vi "config-ICC.vi"() -> ()   [LabVIEW 2024]
uses:
  controls/controller.ctl
  controls/sched-cluster.ctl
  controls/UiScheduleTimestamp.ctl
  controls/UiDeviceSensorParams.ctl
  controls/UiDeviceSensorEquality.ctl
  controls/device-mode.ctl
  controls/UiStepBuilder.ctl
  controls/type.step-builder.ctl
  <vilib>/Utility/miscctls.llb/LVPointTypeDef.ctl
  controls/enumVarCtrlIO.ctl
  controls/enum.io.type.ctl
  controls/enum.io.mode.ctl
  <vilib>/Utility/error.llb/DialogType.ctl
  controls/state-engine.ctl
  <vilib>/Utility/libraryn.llb/Create Directory Recursive.vi
  globals/globals-engine.vi
panel:
  out "procNameID":string
  in  "Ctrl Reload":bool
  in  "Help Page":bool
  in  "Tab Control":enum32{"Main", "Manual Activation", "Help"}(tab)
  in  "Ctrl Save":bool
  in  "Controller":T1={"Schedular"={"sched-mode"=enum."Hourly", "sched-pairs"=[]}, "Sensor"={"Input"="INPUT:", "Comparison"=">=", "Setpoint"=0.0}, "Outputs"=[], "Interval"=0, "Timeout"=1, "Mode"=enum."On"} caption="Device Setup" {"Schedular"."sched-pairs"."start" format="%<%H:%M %d/%m>T"; "Schedular"."sched-pairs"."stop" format="%<%H:%M %d/%m>T"; "Timeout" min=1}
  in  "SEC":u16(ring)=1 caption="Section" items=["H1"]
  in  "Manual.Activation":bool
  in  "DEV":u16(ring)=1 caption="Device" items=["CNETFOG", "CO2", "COOLFAN", "FAC_VENT", "Fan1", "Fan2", "Fan3", "PBRDIGEST", "SCREEN", "WETWALL"]
  in  "Cluster":T7={"Send"=FALSE, "Timeout"=10, "State"=FALSE} {"Timeout" min=1 step=1}
  in  "Manual.Return":bool
  in  "Manual.Return 2":bool
  out "NewDevice":string
  in  "Data Changed?":bool=TRUE
  in  "DEV Reload":bool
  in  "SEC Reload":bool
  out "dir name":string="ICC"
  out "Flow Steps":T8[](array[typedef])
  out "event counter":i32
  in  "DEV Set Strings":bool
  in  "SEC Set Strings":bool
  # "Pulse [sec]"
  # "Period [sec]"
  # "Sensor"
  # "Scheduler"
  # "Note: Timeout value must be above zero."
  # "Indoor Climate Control Configurator\n\nFor devices required pulse activation set \nPulse Width parameter greater then zero (and less then Period).\n\nFor devices required constant ON signal set \nPulse Width parameter greater then Period value."
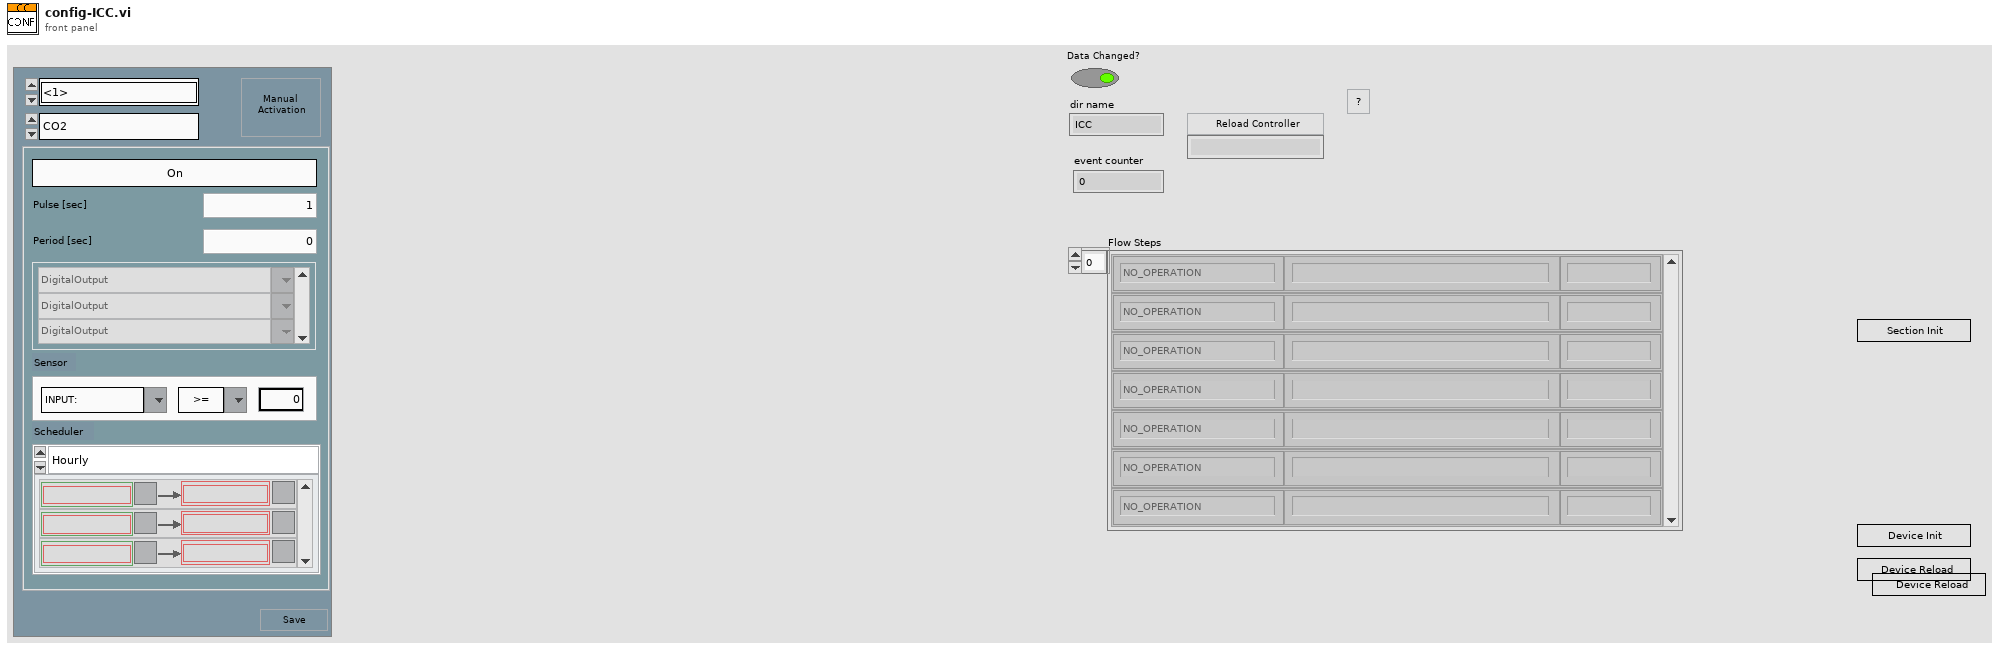
[diagram p1: front panel]
types:
  T1 = typedef "controller.ctl" = cluster{"Schedular":T2, "Sensor":T4, "Outputs":string[], "Interval":u32, "Timeout":u16, "Mode":T6}
  T2 = typedef "sched-cluster.ctl" = cluster{"sched-mode":enum16{"Hourly", "Daily", "Weekly", "Date"}, "sched-pairs":cluster{"start":T3, "stop":T3}[]}
  T3 = typedef "UiScheduleTimestamp.ctl" = timestamp
  T4 = typedef "UiDeviceSensorParams.ctl" = cluster{"Input":string, "Comparison":T5, "Setpoint":dbl}
  T5 = typedef "UiDeviceSensorEquality.ctl" = string
  T6 = typedef "device-mode.ctl" = enum16{"On", "Off", "Sense", "Sched", "Sched AND Sense", "Sched OR Sense"}
  T7 = cluster{"Send":bool, "Timeout":u16, "State":bool}
  T8 = typedef "UiStepBuilder.ctl" = cluster{"Step Function":T9, "ParamString":string, "Step Label":string}
  T9 = typedef "type.step-builder.ctl" = enum16{"NO_OPERATION", "DELAY-JUMP", "DELAY", "JUMP", "COMPLETE", "SCHEDULER", "IRR-CHECK", "UNIT-CHECK", "UNIT-SAMPLE", "UNIT-DOSE", "LOG-REPORT", "LOG-MESSAGE", "IO-READ", "IO-READ-MANY", "IO-WRITE", "IO-COMPARE-OUT", "IO-COMPARE-IN", "PROC-START", "PROC-STOP", "PROC-LOAD", "PROC-IS-COMPLETED", "RECORD-MOVE", "GET-RH", "GET-UV", "GET-WD", "GET-WS", "OCS-CHECK", "OCS-RECORD"}
  T10 = typedef "LVPointTypeDef.ctl" = cluster{"Horizontal":i16, "Vertical":i16}
  T11 = typedef "enum.io.type.ctl" = enum16{"Type", "DI", "DO", "AI", "AO", "VL", "BUF"}
  T12 = typedef "enumVarCtrlIO.ctl" = enum16{"IO Get By Key", "IO List Configs", "IO Add By Key", "IO Modify Value By Key", "IO Modify Calib By Key", "IO Modify ADDR By Key", "IO Modify Mode By Key", "IO Modify Type By Key", "IO Modify Name By Key", "IO Remove By Key", "IO Remove All"}
  T13 = cluster{"state":bool, "timeout":u16, "Name":string}
  T14 = typedef "state-engine.ctl" = enum16{"ENG.NO-OP", "ENG.START", "ENG.STOP", "ENG.EXECUTE", "ENG.STATUS", "ENG.EXTERNAL-CALL", "ENG.INIT", "ENG.INIT.VARS", "ENG.INIT.SERIAL", "ENG.LOAD", "ENG.LOAD.SINGLE", "ENG.LOAD.MODULE", "ENG.LOAD.RELOAD", "ENG.LOAD.UNLOAD", "ENG.IO.LOAD", "ENG.IO.SAVE", "ENG.PROC.RELOAD-BY-NAME", "ENG.PROC.START", "ENG.PROC.STOP", "ENG.PROC.INSERT-STEPS", "ENG.PROC.ISRUNNING", "ENG.PROC.PRESET", "ENG.PROC.STATUS", "ENG.PRINT-USER-MSG", "ENG.RIO.SNAPSHOT", "ENG.RIO.AIN-SNAPSHOT-CALIB", "ENG.RIO.DOUT-BY-ADDR", "ENG.RIO.DOUT-BY-NAME", "ENG.RIO.RFS-DELAY-SET-X1", "ENG.RIO.RFS-DELAY-SET-X8", "ENG.RIO.RFS-CYCLES-SET", "ENG.RIO.RFS-CYCLES-GET", "ENG.RIO.RFS-ENABLE", "ENG.EXIT"}
  T15 = enum32{"Invalid", "Standard", "Closed", "Hidden", "Minimized", "Maximized"}
  T16 = typedef "enum.io.mode.ctl" = enum16{"Mode", "RIO", "SIM"}
  T17 = typedef "IONode.ctl" = cluster{"ADDR":T18, "Label":string, "Type":T11, "Mode":T16, "Value":string, "Tags":string, "calibration":T19[]}
  T18 = typedef "type.address.ctl" = u16
  T19 = typedef "typeXyPoint.ctl" = cluster{"X":dbl, "Y":dbl}
  T20 = typedef "DialogType.ctl" = u16
  T21 = cluster{"Boolean State":bool, "Ch":u8, "Address":u8, "Timeout":u8}
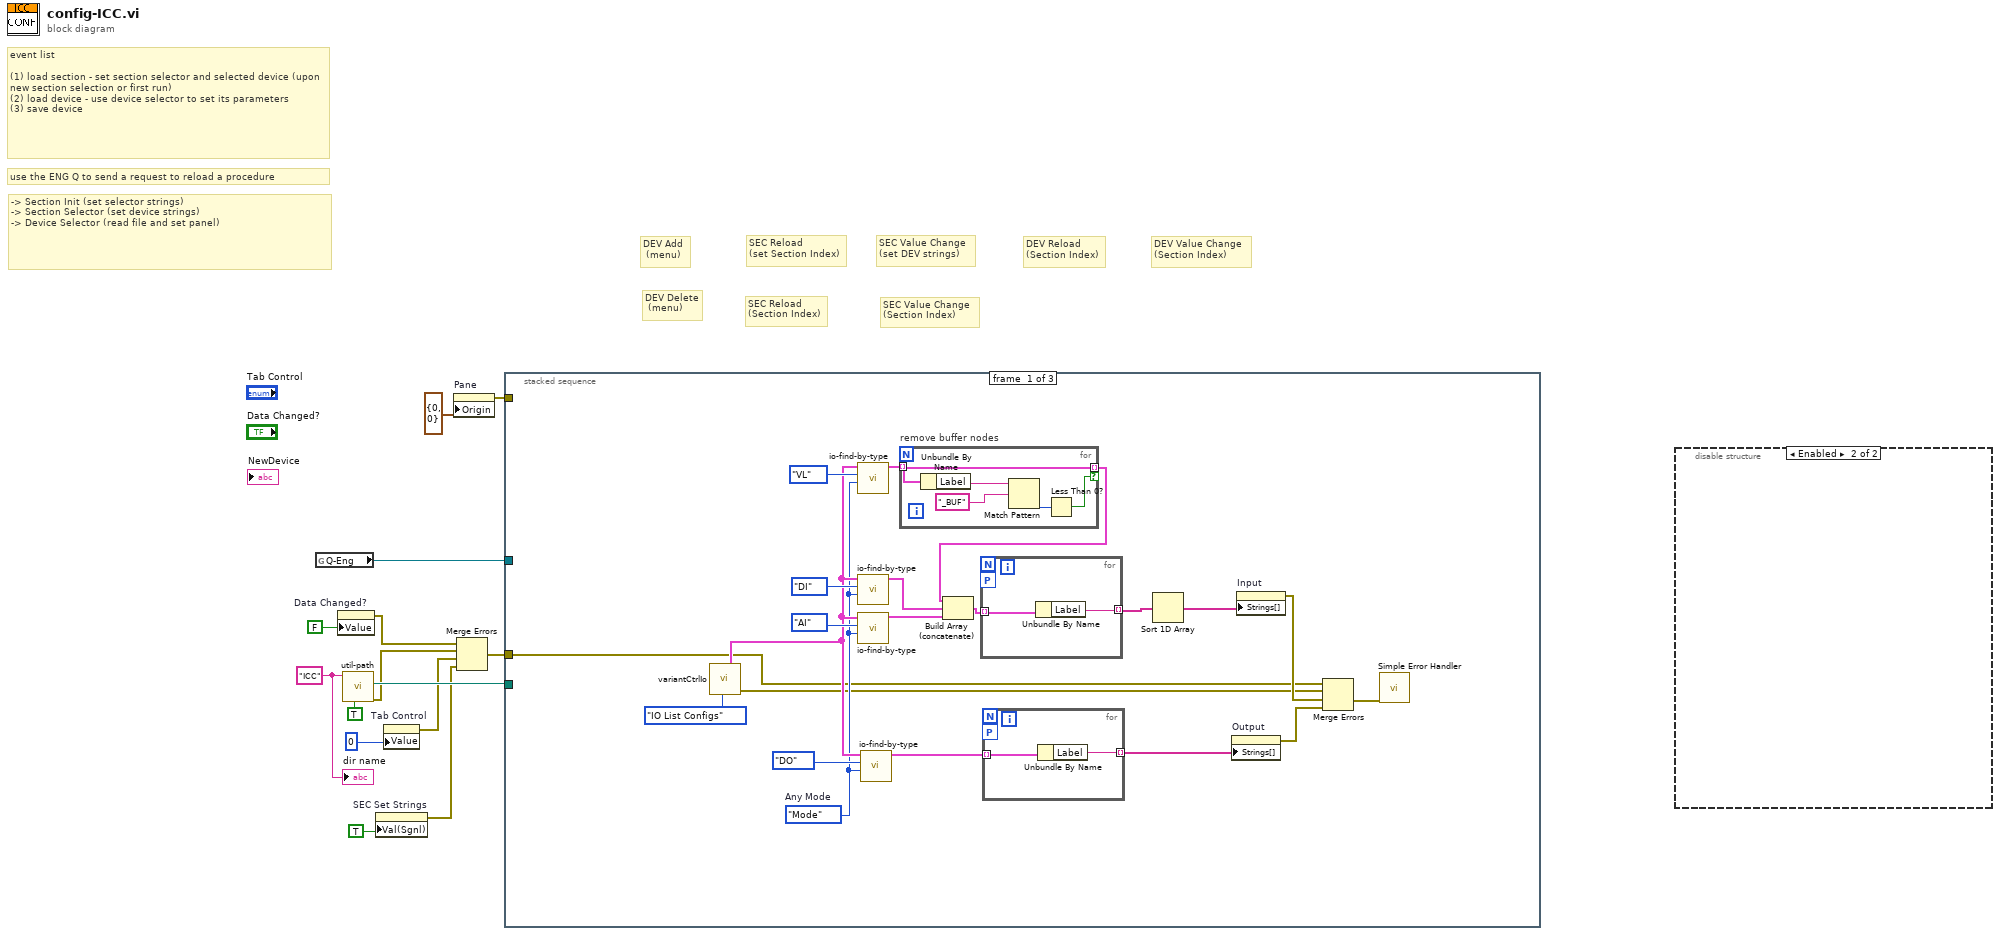
[diagram p0: block diagram]
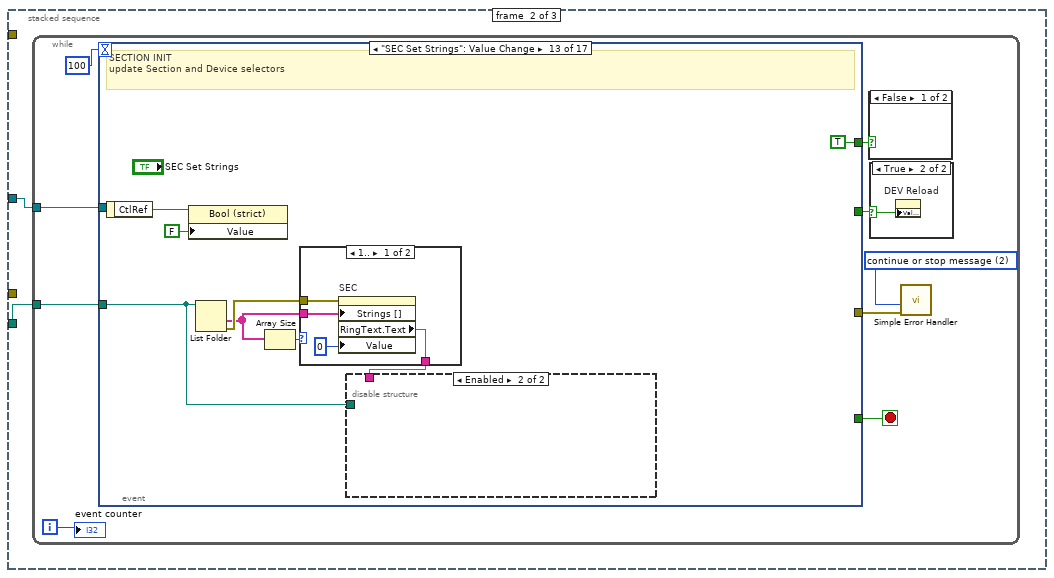
[diagram p3: hidden frame]
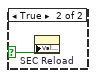
[diagram p5: hidden frame]
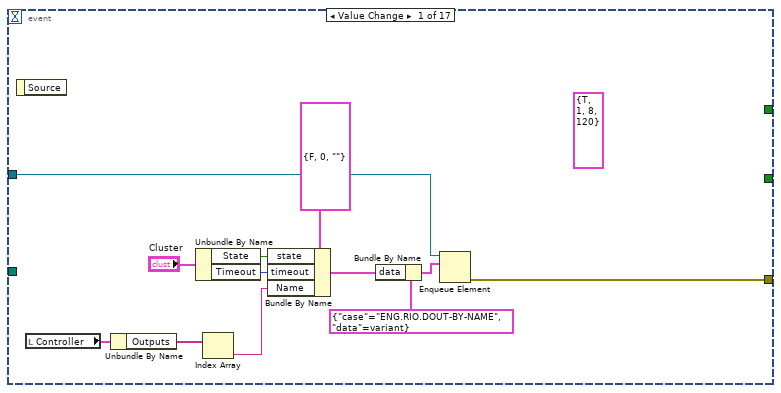
[diagram p6: hidden frame]
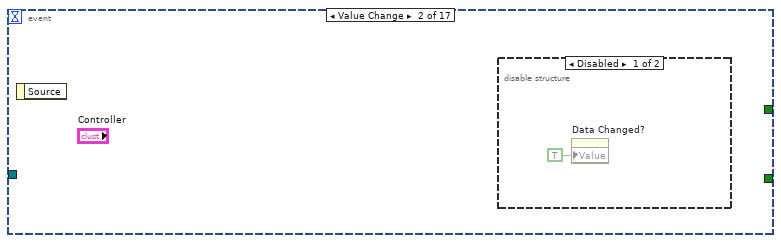
[diagram p7: hidden frame]
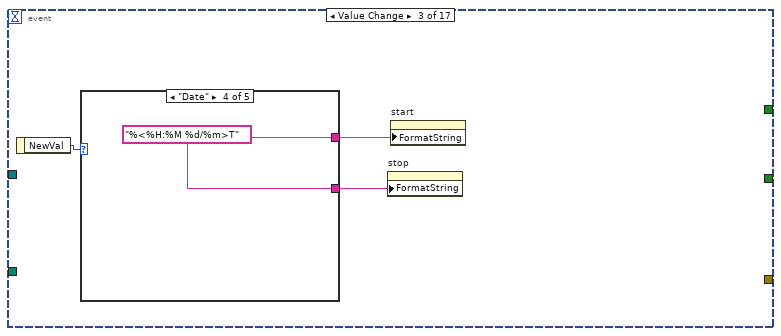
[diagram p9: hidden frame]
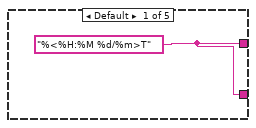
[diagram p10: hidden frame]
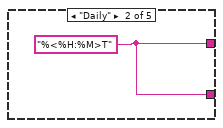
[diagram p11: hidden frame]
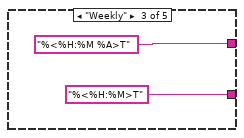
[diagram p12: hidden frame]
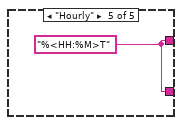
[diagram p13: hidden frame]
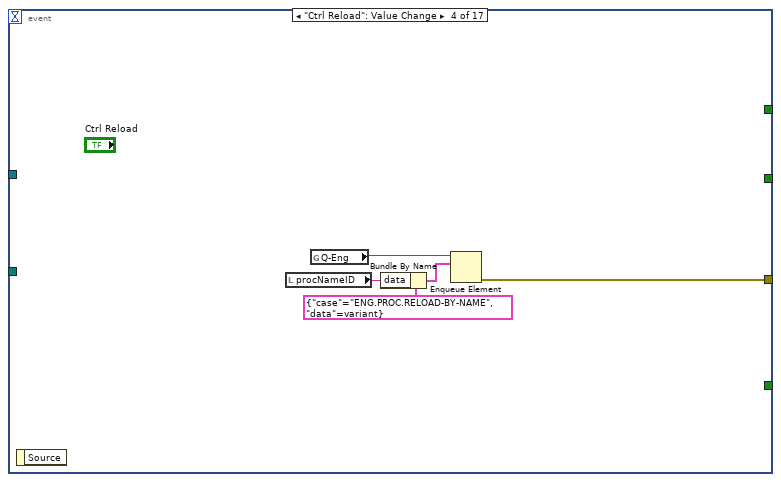
[diagram p14: hidden frame]
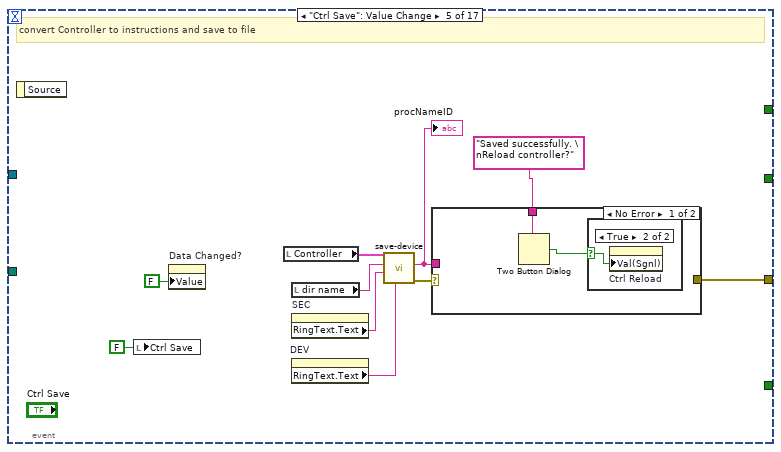
[diagram p15: hidden frame]
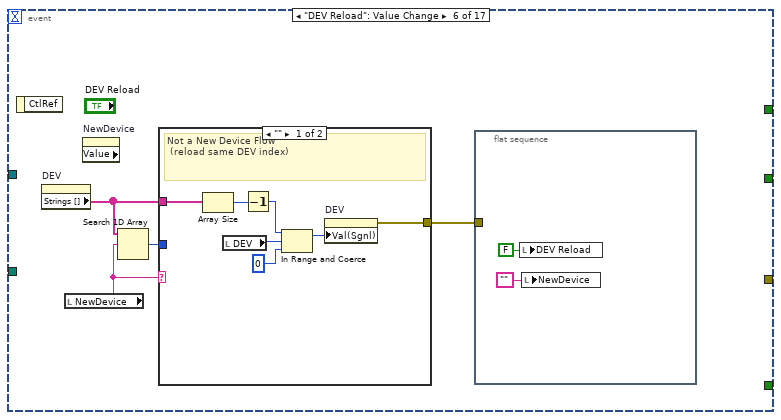
[diagram p18: hidden frame]
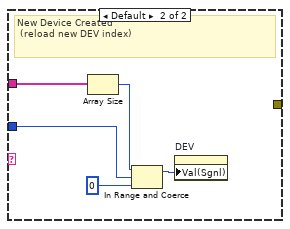
[diagram p19: hidden frame]
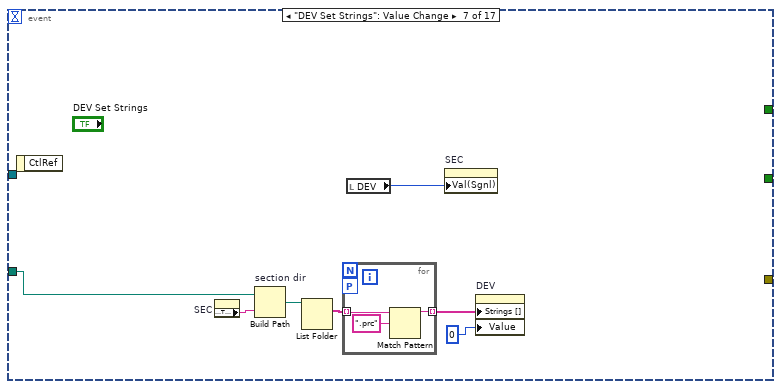
[diagram p20: hidden frame]
diagram:
  w9 = "ICC" ("dir name")
  # "DEV Value Change\n(Section Index)"
  # "SEC Value Change\n(Section Index)"
  # "SEC Reload\n(Section Index)"
  # "DEV Delete\n (menu)"
  # "DEV Reload\n(Section Index)"
  # "DEV Add\n (menu)"
  # "SEC Value Change\n(set DEV strings)"
  # "SEC Reload\n(set Section Index)"
  # "-> Section Init (set selector strings)\n-> Section Selector (set device strings)\n-> Device Selector (read file and set panel)"
  # "use the ENG Q to send a request to reload a procedure"
  # "event list\n\n(1) load section - set section selector and selected device (upon new section selection or first run)\n(2) load device - use device selector to set its parameters \n(3) save device"
  n1 = global read "globals-engine.vi" "Q-Eng"() -> (w7:refnum<queue>)
  n2 = property on="Data Changed?" class="Bool (strict)"("Value"=FALSE ("Data Changed?")) -> (error out=w6:errorcluster)  [unwired: 2 in, 1 out]
  n3 = call "util-path.vi"("Create Folders?(F)"=TRUE, "append path (ie. folder\\filename.*)"=w9) -> ("error out"=w5:errorcluster, "SelectedPath"=w12:path)  [unwired: 5 in, 3 out]
  n4 = property on="SEC Set Strings" class="Bool (strict)"("Val(Sgnl)"=TRUE ("Section Load")) -> (error out=w3:errorcluster)  [unwired: 2 in, 1 out]
  n5 = property on="Tab Control" class="TabCtl (strict)"("Value"=0) -> (error out=w4:errorcluster)  [unwired: 2 in, 1 out]
  n6 = property on="Pane" class="Pane"("Origin"=T10 {"Horizontal"=0, "Vertical"=0}) -> (error out=w13:errorcluster)  [unwired: 2 in, 1 out]
  n7 = Merge Errors(w6, w5, w4, w3) -> (w1:errorcluster)
  n8 = stacked-sequence {
    tunnel: w12 -> [_ w46 _]
    tunnel: w13 -> [_ _ _]
    tunnel: w7 -> [_ w45 _]
    tunnel: w1 -> [w15 _ _]
    frame #0 {
      w23 = enum.io.mode."Mode"  # Any Mode
      n9 = call "variantCtrlIo.vi"("menu (Get Param)"=enumVarCtrlIO."IO List Configs" ("menu (get)")) -> ("error out"=w17:errorcluster, "IO Configs List"=w24:T17[])  [unwired: 6 in, 3 out]
      n10 = call "io-find-by-type.vi"("Mode(Any)"=w23, "Type"=enum.io.type."VL" ("type"), "IOConfigs in"=w24) -> ("Search Results"=w22:T17[])  [unwired: 8 in]
      n11 = call "io-find-by-type.vi"("Mode(Any)"=w23, "Type"=enum.io.type."DI" ("type"), "IOConfigs in"=w24) -> ("Search Results"=w32:T17[])  [unwired: 8 in]
      n12 = call "io-find-by-type.vi"("Mode(Any)"=w23, "Type"=enum.io.type."AI" ("type"), "IOConfigs in"=w24) -> ("Search Results"=w31:T17[])  [unwired: 8 in]
      n13 = call "io-find-by-type.vi"("Mode(Any)"=w23, "Type"=enum.io.type."DO" ("type"), "IOConfigs in"=w24) -> ("Search Results"=w27:T17[])  [unwired: 8 in]
      n14 = for "remove buffer nodes" {
        tunnel: w22 -> [w37] mode=indexing
        tunnel: [w37] -> w21 mode=indexing if=w36
        n15 = Unbundle By Name(w37) -> ("Label"=w40:string)
        n16 = Match Pattern(string=w40, regular expression="_BUF") -> (offset past match=w38:i32)  [unwired: 1 in, 3 out]
        n17 = Less Than 0?(x=w38) -> (x < 0?=w36:bool)
      }
      n18 = Build Array (concatenate)(w21, w32, w31) -> (w30:T17[])
      n19 = for {
        tunnel: w30 -> [w44] mode=indexing
        tunnel: [w43] -> w35 mode=indexing
        workers-P: _ -> [_]
        n20 = Unbundle By Name(w44) -> ("Label"=w43:string)
      }
      n21 = for {
        tunnel: w27 -> [w42] mode=indexing
        tunnel: [w41] -> w26 mode=indexing
        workers-P: _ -> [_]
        n22 = Unbundle By Name(w42) -> ("Label"=w41:string)
      }
      n23 = Sort 1D Array(array=w35) -> (sorted array=w20:string[])
      n24 = property on="Output" class="CmbBox"("Strings[]"=w26) -> (error out=w18:errorcluster)  [unwired: 2 in, 1 out]
      n25 = property on="Input" class="CmbBox"("Strings[]"=w20) -> (error out=w19:errorcluster)  [unwired: 2 in, 1 out]
      n26 = Merge Errors(w15, w17, w19, w18) -> (w16:errorcluster)
      n27 = call <vilib>:"Simple Error Handler.vi"("error in (no error)"=w16) -> ()  [unwired: 4 in, 5 out]
    }
    frame #1 {
      n28 = while {
        tunnel: w46 -> [w54]
        tunnel: w45 -> [w47]
        i -> [w53]
        stop <- w55 stop-if-true
        w51 = T20 2 items=["no dialog", "OK message", "continue or stop message", "OK message + warnings", "continue/stop + warnings"] ("type of dialog (OK msg:1)")
        n29 = event shown="[12] \"SEC Set Strings\": Value Change" {
          selector: _ -> [_ _ _ _ _ _ _ _ _ _ _ _ _ _ _ _ _]
          dyn-events: _ -> [_ _ _ _ _ _ _ _ _ _ _ _ _ _ _ _ _]
          timeout: 100 -> [_ _ _ _ _ _ _ _ _ _ _ _ _ _ _ _ _]
          tunnel: [_ _ _ _ _ _ _ _ _ _ _ _ _ _ FALSE w356 w363] -> w55
          tunnel: w54 -> [_ _ _ _ _ _ w117 _ _ _ _ _ w170 w191 w218 _ _]
          tunnel: [w61 _ _ w80 w88 _ _ w128 _ _ _ _ _ _ w216 _ _] -> w52
          tunnel: [_ _ _ _ _ _ _ _ _ _ _ _ TRUE _ w217 _ _] -> w50
          tunnel: [_ _ _ _ _ _ _ _ _ _ _ _ _ w189 _ _ _] -> w49
          tunnel: w47 -> [w58 _ _ _ _ _ _ _ _ _ _ _ _ _ w214 _ _]
          event "Cluster.Send": Value Change {
            (unwired) T21 {"Boolean State"=TRUE, "Ch"=1, "Address"=8, "Timeout"=120} ("digitalPort")
            n30 = event-data() -> ()  [unwired: 1 in, 1 out]
            n31 = local read "Controller"() -> (w62:T1)
            n32 = Unbundle By Name(w62) -> ("Outputs"=w60:string[])
            n33 = Unbundle By Name("Cluster") -> ("State"=w64:bool, "Timeout"=w63:u16)
            n34 = Index Array(array=w60) -> (element=w59:string)  [unwired: 1 in]
            n35 = Bundle By Name(cluster=T13 {"state"=FALSE, "timeout"=0, "Name"=""} ("Cluster"), "state"=w64, "timeout"=w63, "Name"=w59) -> (w66:T13)
            n36 = Bundle By Name(cluster=cluster{"case":T14, "data":variant} {"case"=enum."ENG.RIO.DOUT-BY-NAME", "data"=variant} ("element"), "data"=w66) -> (w68:cluster{"case":T14, "data":variant})
            n37 = Enqueue Element(queue=w58, element=w68) -> (error out=w61:errorcluster)  [unwired: 2 in, 2 out]
          }
          event Value Change {
            n38 = event-data() -> ()  [unwired: 1 in, 1 out]
            n39 = disable-structure shown="Disabled" {
              frame Disabled {
                n40 = property on="Data Changed?" class="Bool (strict)"("Value"=TRUE ("Data Changed?")) -> ()  [unwired: 2 in, 2 out]
              }
              frame Enabled {
              }
            }
          }
          event Value Change {
            n41 = event-data() -> ("NewVal"=w73:enum16{"Hourly", "Daily", "Weekly", "Date"})  [unwired: 1 in]
            n42 = case shown="\"Date\"" w73 {
              tunnel: [w74 w75 "%<%H:%M %A>T" ("Format String") w78 w79] -> w72
              tunnel: [w74 w75 "%<%H:%M>T" ("Format String") w78 w79] -> w71
              frame Default {
                w74 = "%<%H:%M %d/%m>T" ("Format String")
              }
              frame "Daily" {
                w75 = "%<%H:%M>T" ("Format String")
              }
              frame "Weekly" {
              }
              frame "Date" {
                w78 = "%<%H:%M %d/%m>T" ("Format String")
              }
              frame "Hourly" {
                w79 = "%<HH:%M>T" ("Format String")
              }
            }
            n43 = property on="stop" class="AbsTime (strict)"("FormatString"=w71) -> ()  [unwired: 2 in, 2 out]
            n44 = property on="start" class="AbsTime (strict)"("FormatString"=w72) -> ()  [unwired: 2 in, 2 out]
          }
          event "Ctrl Reload": Value Change {
            n45 = event-data() -> ()  [unwired: 1 in, 1 out]
            n46 = local read "procNameID"() -> (w81:string)
            n47 = global read "globals-engine.vi" "Q-Eng"() -> (w84:refnum<queue>)
            n48 = Bundle By Name(cluster=cluster{"case":T14, "data":variant} {"case"=enum."ENG.PROC.RELOAD-BY-NAME", "data"=variant} ("element"), "data"=w81) -> (w83:cluster{"case":T14, "data":variant})
            n49 = Enqueue Element(queue=w84, element=w83) -> (error out=w80:errorcluster)  [unwired: 2 in, 2 out]
          }
          event "Ctrl Save": Value Change {
            # "convert Controller to instructions and save to file"
            n50 = event-data() -> ()  [unwired: 1 in, 1 out]
            n51 = local write "Ctrl Save"(FALSE ("Ctrl Save")) -> ()
            n52 = property on="Data Changed?" class="Bool (strict)"("Value"=FALSE ("Data Changed?")) -> ()  [unwired: 2 in, 2 out]
            n53 = local read "Controller"() -> (w90:T1)
            n54 = local read "dir name"() -> (w91:string)
            n55 = property on="SEC" class="Ring (strict)"() -> ("RingText.Text"=w93:string)  [unwired: 2 in, 2 out]
            n56 = property on="DEV" class="Ring (strict)"() -> ("RingText.Text"=w92:string)  [unwired: 2 in, 2 out]
            n57 = call "save-device.vi"("Proc Name"=w92, "Module Name"=w93, "Base Folder"=w91, "Device"=w90) -> ("error out"=w89:errorcluster, "procNameID"=w85:string)  [unwired: 6 in]
            "procNameID" <- w85
            n58 = case shown="No Error" w89 {
              selector: w89 -> [_ w98]
              tunnel: w85 -> [_ _]
              tunnel: [_ w98] -> w88
              tunnel: "Saved successfully. \nReload controller?" ("message") -> [w96 _]
              frame No Error {
                n59 = Two Button Dialog(message=w96) -> (T button?=w95:bool)  [unwired: 2 in]
                n60 = case shown="True" w95 {
                  selector: w95 -> [_ w97]
                  frame False {
                  }
                  frame True {
                    n61 = property on="Ctrl Reload" class="Bool (strict)"("Val(Sgnl)"=w97) -> ()  [unwired: 2 in, 2 out]
                  }
                }
              }
              frame Error {
              }
            }
          }
          event "DEV Reload": Value Change {
            n62 = event-data() -> ()  [unwired: 1 in, 1 out]
            n63 = property on="DEV" class="Ring (strict)"() -> ("Strings []"=w102:string[])  [unwired: 2 in, 2 out]
            n64 = local read "NewDevice"() -> (w101:string)
            n65 = property on="NewDevice" class="Str" props=["Value"]() -> ()  [unwired: 2 in, 3 out]
            n66 = Search 1D Array(1D array=w102, element=w101) -> (index of element=w100:i32)  [unwired: 1 in]
            n67 = case shown="\"\"" w101 {
              tunnel: w102 -> [w107 w113]
              tunnel: w100 -> [_ w112]
              tunnel: [w106 _] -> w99
              frame "" {
                # "Not a New Device Flow\n (reload same DEV index)"
                n68 = Array Size(array=w107) -> (size(s)=w110:i32)
                n69 = local read "DEV"() -> (w109:u16)
                n70 = Decrement(x=w110) -> (x-1=w105:i32)
                n71 = In Range and Coerce(upper limit=w105, x=w109, lower limit=0) -> (coerced(x)=w108:i32)  [unwired: 1 out]
                n72 = property on="DEV" class="Ring (strict)"("Val(Sgnl)"=w108) -> (error out=w106:errorcluster)  [unwired: 2 in, 1 out]
              }
              frame Default {
                # "New Device Created\n (reload new DEV index)"
                n73 = Array Size(array=w113) -> (size(s)=w115:i32)
                n74 = In Range and Coerce(upper limit=w115, x=w112, lower limit=0) -> (coerced(x)=w114:i32)  [unwired: 1 out]
                n75 = property on="DEV" class="Ring (strict)"("Val(Sgnl)"=w114) -> ()  [unwired: 2 in, 2 out]
              }
            }
            n76 = flat-sequence {
              tunnel: w99 -> [_]
              frame #0 {
                n77 = local write "DEV Reload"(FALSE ("SEC reload")) -> ()
                n78 = local write "NewDevice"("" ("NewDevice")) -> ()
              }
            }
          }
          event "DEV Set Strings": Value Change {
            n79 = event-data() -> ()  [unwired: 1 in, 1 out]
            n80 = property on="SEC" class="Ring (strict)"() -> ("RingText.Text"=w122:string)  [unwired: 2 in, 2 out]
            n81 = Build Path "section dir"(base path=w117, name or relative path=w122) -> (appended path=w121:path)
            n82 = List Folder(path=w121) -> (filenames=w120:string[])  [unwired: 3 in, 3 out]
            n83 = for {
              tunnel: w120 -> [w126] mode=indexing
              tunnel: [w124] -> w119 mode=indexing
              workers-P: _ -> [_]
              n84 = Match Pattern(string=w126, regular expression=".prc") -> (before substring=w124:string)  [unwired: 1 in, 3 out]
            }
            n85 = local read "DEV"() -> (w123:u16)
            n86 = property on="SEC" class="Ring (strict)"("Val(Sgnl)"=w123) -> ()  [unwired: 2 in, 2 out]
            n87 = property on="DEV" class="Ring (strict)"("Strings []"=w119, "Value"=u16 0 ("Value (Signaling)")) -> ()  [unwired: 2 in, 2 out]
          }
          event "DEV": Value Change {
            n88 = event-data() -> ("OldVal"=w127:u16)  [unwired: 1 in]
            n89 = stacked-sequence {
              seq-local: [w129 _] -> [_ w135]
              tunnel: [_ w136] -> w128
              tunnel: w127 -> [_ w134]
              frame #0 {
                n90 = property on="Data Changed?" class="Bool (strict)"() -> ("Value"=w130:bool)  [unwired: 2 in, 2 out]
                n91 = case shown="False" w130 {
                  tunnel: [TRUE ("T button?") w132] -> w129
                  frame False {
                  }
                  frame True {
                    n92 = Two Button Dialog(message="Proceed without saving?") -> (T button?=w132:bool)  [unwired: 2 in]
                  }
                }
              }
              frame #1 {
                n93 = case shown="True" w135 {
                  tunnel: [_ w144] -> w136
                  tunnel: w134 -> [w137 _]
                  frame False {
                    n94 = local write "DEV"(w137) -> ()
                  }
                  frame True {
                    n95 = local read "dir name"() -> (w142:string)
                    n96 = property on="SEC" class="Ring (strict)"() -> ("RingText.Text"=w141:string)  [unwired: 2 in, 2 out]
                    n97 = property on="DEV" class="Ring (strict)"() -> ("RingText.Text"=w140:string)  [unwired: 2 in, 2 out]
                    n98 = property on="Data Changed?" class="Bool (strict)"("Value"=FALSE ("Data Changed?")) -> ()  [unwired: 2 in, 2 out]
                    n99 = call "clm.config.build-path.vi"("Proc Name"=w140, "Section Name"=w141, "Module Name"=w142) -> ("Relative Path"=w139:string)  [unwired: 8 in]
                    n100 = Empty String/Path?(string/path=w139) -> (empty?=w143:bool)
                    n101 = case shown="False" w143 {
                      tunnel: w139 -> [w153 _]
                      tunnel: [w148 _] -> w144
                      frame False {
                        n102 = call "util.file.vars.vi"("Operation(Read)"=enum16{"Read File", "Write File"}."Read File", "Proc Name(open dialog if empty)"=w153) -> ("error out"=w151:errorcluster, "Vars[] out"=w154:variant[])  [unwired: 5 in, 3 out]
                        n103 = call "build.proc.parse.vi"("error"=w151, "Array in"=w154) -> ("error out"=w150:errorcluster, "Flow Steps"=w149:T8[])  [unwired: 7 in, 1 out]
                        "Flow Steps" <- w149
                        n104 = call "clm.build.flow.parse.vi"("Device Flow"=w149) -> ("error out"=w147:errorcluster, "Device Conf"=w146:T1)  [unwired: 9 in]
                        n105 = Unbundle By Name(w146) -> ("Schedular.sched-mode"=w145:enum16{"Hourly", "Daily", "Weekly", "Date"})
                        n106 = property on="sched-mode" class="Enum (strict)"("Val(Sgnl)"=w145) -> ()  [unwired: 2 in, 2 out]
                        n107 = local write "Controller"(w146) -> ()
                        n108 = Merge Errors(w150, w147) -> (w148:errorcluster)
                      }
                      frame True {
                        # "empty string"
                      }
                    }
                  }
                }
              }
            }
          }
          event "Help Page": Value Change {
            n109 = event-data() -> ()  [unwired: 1 in, 1 out]
            n110 = property on="Tab Control" class="TabCtl (strict)"("Value"=2) -> ()  [unwired: 2 in, 2 out]
          }
          event "Manual.Activation": Value Change {
            n111 = event-data() -> ()  [unwired: 1 in, 1 out]
            n112 = property on="Timeout" class="DigNum (strict)"("Key Focus"=TRUE) -> (error out=w156:errorcluster)  [unwired: 2 in, 1 out]
            n113 = property on="Tab Control" class="TabCtl (strict)"(error in=w156, "Value"=1) -> ()  [unwired: 1 in, 2 out]
          }
          event "Manual.Return", "Manual.Return 2": Value Change {
            n114 = event-data() -> ()  [unwired: 1 in, 1 out]
            n115 = property on="Tab Control" class="TabCtl (strict)"("Value"=0) -> ()  [unwired: 2 in, 2 out]
          }
          event "SEC Reload": Value Change {
            n116 = event-data() -> ()  [unwired: 1 in, 1 out]
            n117 = property on="SEC" class="Ring (strict)"() -> ("Strings []"=w162:string[])  [unwired: 2 in, 2 out]
            n118 = local write "SEC Reload"(FALSE ("SEC reload")) -> ()
            n119 = local read "SEC"() -> (w164:u16)
            n120 = Array Size(array=w162) -> (size(s)=w161:i32)
            n121 = In Range and Coerce(upper limit=w161, x=w164, lower limit=0) -> (coerced(x)=w163:i32)  [unwired: 1 out]
            n122 = property on="SEC" class="Ring (strict)"("Val(Sgnl)"=w163) -> ()  [unwired: 2 in, 2 out]
          }
          event "SEC Set Strings": Value Change {
            # "SECTION INIT\nupdate Section and Device selectors"
            n123 = event-data() -> ("CtlRef"=w172:refnum<vi>)  [unwired: 1 in]
            n124 = property class="Bool (strict)"(reference=w172, "Value"=FALSE) -> ()  [unwired: 1 in, 2 out]
            n125 = List Folder(path=w170) -> (folder names=w168:string[], error out=w173:errorcluster)  [unwired: 3 in, 2 out]
            n126 = Array Size(array=w168) -> (size(s)=w167:i32)
            n127 = case shown="1.." w167 {
              tunnel: w168 -> [w177 w179]
              tunnel: w173 -> [w176 w178]
              tunnel: [w175 _] -> w169
              frame 1.. {
                n128 = property on="SEC" class="Ring (strict)"(error in=w176, "Strings []"=w177, "Value"=0) -> ("RingText.Text"=w175:string)  [unwired: 1 in, 2 out]
              }
              frame 0, Default {
                # "no sections defined"
                n129 = property on="SEC" class="Ring (strict)"(error in=w178, "Strings []"=w179) -> ()  [unwired: 1 in, 2 out]
              }
            }
            n130 = disable-structure shown="Enabled" {
              disable-tunnel: w170 -> [w185 _]
              disable-tunnel: w169 -> [w184 _]
              frame Disabled {
                n131 = Build Path "section dir"(base path=w185, name or relative path=w184) -> (appended path=w183:path)
                n132 = List Folder(path=w183) -> (filenames=w181:string[])  [unwired: 3 in, 3 out]
                n133 = for {
                  tunnel: w181 -> [w188] mode=indexing
                  tunnel: [w186] -> w180 mode=indexing
                  n134 = Match Pattern(string=w188, regular expression=".prc") -> (before substring=w186:string)  [unwired: 1 in, 3 out]
                }
                n135 = property on="Schedular" class="Clust (strict)"("Strings []"=w180, "Val(Sgnl)"=u16 0 ("Value (Signaling)")) -> ()  [unwired: 2 in, 2 out]
              }
              frame Enabled {
              }
            }
          }
          event "SEC": Value Change {
            # "SECTION SELECTOR - VALUE CHANGE\nLoad Device Selector using the new Section Selector"
            n136 = event-data() -> ("OldVal"=w190:u16)  [unwired: 1 in]
            n137 = stacked-sequence {
              seq-local: [w192 _] -> [_ w199]
              tunnel: w191 -> [_ w200]
              tunnel: w190 -> [_ w198]
              tunnel: [_ w197] -> w189
              frame #0 {
                n138 = property on="Data Changed?" class="Bool (strict)"() -> ("Value"=w193:bool)  [unwired: 2 in, 2 out]
                n139 = case shown="False" w193 {
                  tunnel: [TRUE ("T button?") w195] -> w192
                  frame False {
                  }
                  frame True {
                    n140 = Two Button Dialog(message="Proceed without saving?") -> (T button?=w195:bool)  [unwired: 2 in]
                  }
                }
              }
              frame #1 {
                n141 = case shown="True" w199 {
                  tunnel: w200 -> [_ w206]
                  tunnel: w198 -> [w201 _]
                  tunnel: [_ TRUE] -> w197
                  frame False {
                    n142 = local write "SEC"(w201) -> ()
                  }
                  frame True {
                    n143 = property on="SEC" class="Ring (strict)"() -> ("RingText.Text"=w210:string)  [unwired: 2 in, 2 out]
                    n144 = Build Path "section dir"(base path=w206, name or relative path=w210) -> (appended path=w209:path)
                    n145 = List Folder(path=w209) -> (filenames=w208:string[], error out=w203:errorcluster)  [unwired: 3 in, 2 out]
                    n146 = call <vilib>:"Clear Errors.vi"("error in (no error)"=w203, "specific error code to clear (0: all)"=1430) -> ()  [unwired: 4 in, 2 out]
                    n147 = property on="Data Changed?" class="Bool (strict)"("Value"=FALSE ("Data Changed?")) -> ()  [unwired: 2 in, 2 out]
                    n148 = for {
                      tunnel: w208 -> [w213] mode=indexing
                      tunnel: [w211] -> w207 mode=indexing
                      workers-P: _ -> [_]
                      n149 = Match Pattern(string=w213, regular expression=".prc") -> (before substring=w211:string)  [unwired: 1 in, 3 out]
                    }
                    n150 = property on="DEV" class="Ring (strict)"("Strings []"=w207) -> ()  [unwired: 2 in, 2 out]
                  }
                }
              }
            }
          }
          event Menu Selection (User) {
            n151 = event-data() -> ("ItemTag"=w219:string)  [unwired: 1 in, 1 out]
            n152 = case shown="\"DEV_ADD\"" w219 {
              tunnel: w218 -> [_ _ w263 _ w286 w297 w323 _]
              tunnel: [TRUE w234 w259 _ _ _ w319 _] -> w217
              tunnel: [w224 w233 w258 _ w285 w296 w318 _] -> w216
              tunnel: w214 -> [_ _ _ _ _ _ _ _]
              frame "DEV_ADD" {
                n153 = call "ui-form-text-line.vi"("User Prompt in"="Please provide a name for the new device") -> ("Cancelled?"=w222:bool, "text out"=w221:string)  [unwired: 9 in]
                n154 = case shown="False" w222 {
                  tunnel: [w227 _] -> w224
                  tunnel: w221 -> [w226 _]
                  tunnel: [w226 _] -> w220
                  frame False {
                    # "Not Cancelled"
                    n155 = property on="SEC" class="Ring (strict)"() -> ("RingText.Text"=w230:string)  [unwired: 2 in, 2 out]
                    n156 = local read "dir name"() -> (w229:string)
                    n157 = call "save-device.vi"("Proc Name"=w226, "Module Name"=w230, "Base Folder"=w229, "Device"=T1 {"Schedular"={"sched-mode"=enum."Hourly", "sched-pairs"=[]}, "Sensor"={"Input"="", "Comparison"="", "Setpoint"=0.0}, "Outputs"=[], "Interval"=60, "Timeout"=0, "Mode"=enum."Off"} ("Device 2")) -> ("error out"=w227:errorcluster)  [unwired: 6 in, 1 out]
                  }
                  frame True {
                  }
                }
                n158 = local write "NewDevice"(w220) -> ()
              }
              frame "DEV_DELETE" {
                n159 = property on="SEC" class="Ring (strict)"() -> ("RingText.Text"=w243:string)  [unwired: 2 in, 2 out]
                n160 = property on="DEV" class="Ring (strict)"() -> ("RingText.Text"=w242:string)  [unwired: 2 in, 2 out]
                n161 = local read "dir name"() -> (w244:string)
                n162 = Concatenate Strings(w242, ".*" ("string")) -> (w241:string)
                n163 = call "clm.config.build-path.vi"("Proc Name"=w241, "Section Name"=w243, "Module Name"=w244) -> ("Relative Path"=w240:string)  [unwired: 8 in]
                n164 = call "util-path.vi"("append path (ie. folder\\filename.*)"=w240) -> ("error out"=w250:errorcluster, "SelectedPath"=w248:path, ".extension (.prc)"=w246:string)  [unwired: 6 in, 2 out]
                n165 = Strip Path(path=w248) -> (name=w247:string)  [unwired: 1 out]
                n166 = Search and Replace String(input string=w247, search string=w246) -> (result string=w245:string)  [unwired: 6 in, 3 out]
                n167 = Format Into String(format string="Delete %s?", w245) -> (resulting string=w232:string)  [unwired: 2 in, 1 out]
                n168 = Two Button Dialog(message=w232) -> (T button?=w231:bool)  [unwired: 2 in]
                n169 = case shown="True" w231 {
                  tunnel: w250 -> [w252 w257]
                  tunnel: [w252 w256] -> w249
                  tunnel: w248 -> [_ w255]
                  tunnel: [TRUE ("cancelled") w254] -> w239
                  frame False {
                  }
                  frame True {
                    n170 = Delete(path (use dialog)=w255, confirm (F)=FALSE, error in=w257) -> (cancelled=w254:bool, error out=w256:errorcluster)  [unwired: 2 in, 1 out]
                  }
                }
                n171 = call <vilib>:"Clear Errors.vi"("error in (no error)"=w249, "specific error code to clear (0: all)"=43) -> ("error out"=w233:errorcluster)  [unwired: 4 in, 1 out]
                n172 = Compound Arithmetic op=AND(TRUE, invert w239) -> (w234:bool)
              }
              frame "DEV_RENAME" {
                n173 = call "ui-form-text-line.vi"("User Prompt in"="Enter Device Name:") -> ("Cancelled?"=w261:bool, "text out"=w262:string)  [unwired: 9 in]
                n174 = case shown="False" w261 {
                  tunnel: w262 -> [w271 _]
                  tunnel: w263 -> [_ _]
                  tunnel: [w265 _] -> w259
                  tunnel: [w264 _] -> w258
                  frame False {
                    # "Not Canceled"
                    n175 = property on="DEV" class="Ring (strict)"() -> ("RingText.Text"=w281:string)  [unwired: 2 in, 2 out]
                    n176 = property on="SEC" class="Ring (strict)"() -> ("RingText.Text"=w282:string)  [unwired: 2 in, 2 out]
                    n177 = property on="SEC" class="Ring (strict)"() -> ("RingText.Text"=w275:string)  [unwired: 2 in, 2 out]
                    n178 = local read "dir name"() -> (w283:string)
                    n179 = local read "dir name"() -> (w274:string)
                    n180 = Concatenate Strings(w271, ".*" ("string")) -> (w276:string)
                    n181 = Concatenate Strings(w281, ".*" ("string")) -> (w280:string)
                    n182 = call "clm.config.build-path.vi"("Proc Name"=w280, "Section Name"=w282, "Module Name"=w283) -> ("Relative Path"=w273:string)  [unwired: 8 in]
                    n183 = call "clm.config.build-path.vi"("Proc Name"=w276, "Section Name"=w275, "Module Name"=w274) -> ("Relative Path"=w270:string)  [unwired: 8 in]
                    n184 = call "util-path.vi"("append path (ie. folder\\filename.*)"=w273) -> ("error out"=w268:errorcluster, "SelectedPath"=w272:path)  [unwired: 6 in, 3 out]
                    n185 = call "util-path.vi"("append path (ie. folder\\filename.*)"=w270) -> ("error out"=w267:errorcluster, "SelectedPath"=w269:path)  [unwired: 6 in, 3 out]
                    n186 = Merge Errors(w268, w267) -> (w266:errorcluster)
                    n187 = Move(source path=w272, error in=w266, 10:w269) -> (error out=w264:errorcluster)  [unwired: 2 in, 2 out]
                    n188 = Compound Arithmetic op=AND(TRUE ("Value (Signaling)"), invert w264) -> (w265:bool)
                  }
                  frame True {
                    # "Cancelled"
                  }
                }
              }
              frame "DEV_SAVE" {
                n189 = property on="Ctrl Save" class="Bool (strict)"("Val(Sgnl)"=TRUE ("Value (Signaling)")) -> ()  [unwired: 2 in, 2 out]
              }
              frame "SEC_ADD" {
                n190 = call "ui-form-text-line.vi"("User Prompt in"="Enter Section name.") -> ("Cancelled?"=w288:bool, "text out"=w289:string)  [unwired: 9 in]
                n191 = case shown="False" w288 {
                  tunnel: w289 -> [w294 _]
                  tunnel: w286 -> [w295 _]
                  tunnel: [w293 _] -> w285
                  frame False {
                    # "Continue"
                    n192 = Build Path(base path=w295, name or relative path=w294) -> (appended path=w292:path)
                    n193 = Create Folder(path (use dialog)=w292) -> (error out=w291:errorcluster)  [unwired: 2 in, 2 out]
                    n194 = property on="SEC Set Strings" class="Bool (strict)"(error in=w291, "Val(Sgnl)"=TRUE ("Value (Signaling)")) -> (error out=w293:errorcluster)  [unwired: 1 in, 1 out]
                  }
                  frame True {
                    # "Cancelled"
                  }
                }
              }
              frame "SEC_DELETE" {
                n195 = property on="SEC" class="Ring (strict)"() -> ("RingText.Text"=w305:string)  [unwired: 2 in, 2 out]
                n196 = Build Path(base path=w297, name or relative path=w305) -> (appended path=w303:path)
                n197 = List Folder(path=w303) -> (filenames=w302:string[], error out=w300:errorcluster)  [unwired: 3 in, 2 out]
                n198 = Array Size(array=w302) -> (size(s)=w301:i32)
                n199 = Format Into String(format string="Delete section %s with %d devices?" ("User Prompt in"), error in=w300, w305, w301) -> (resulting string=w304:string, error out=w299:errorcluster)  [unwired: 1 in]
                n200 = case shown="No Error" w299 {
                  selector: w299 -> [_ w317]
                  tunnel: w304 -> [w306 _]
                  tunnel: [w308 w317] -> w296
                  tunnel: w303 -> [w307 _]
                  frame No Error {
                    n201 = Two Button Dialog(message=w306, 2:"Delete" ("T button name (\"OK\")")) -> (T button?=w309:bool)  [unwired: 1 in]
                    n202 = case shown="True" w309 {
                      tunnel: w307 -> [_ w316]
                      tunnel: [_ w311] -> w308
                      frame False {
                      }
                      frame True {
                        n203 = Delete(path (use dialog)=w316, entire hierarchy (F)=TRUE, confirm (F)=FALSE) -> (error out=w312:errorcluster)  [unwired: 2 in, 2 out]
                        n204 = property on="SEC Set Strings" class="Bool (strict)"(error in=w312, "Val(Sgnl)"=TRUE ("Value (Signaling)")) -> (error out=w311:errorcluster)  [unwired: 1 in, 1 out]
                      }
                    }
                  }
                  frame Error {
                  }
                }
              }
              frame "SEC_DUPLICATE" {
                n205 = call "ui-form-text-line.vi"("User Prompt in"="Enter new section name:") -> ("Cancelled?"=w321:bool, "text out"=w322:string)  [unwired: 9 in]
                n206 = case shown="False" w321 {
                  tunnel: w322 -> [w324 _]
                  tunnel: w323 -> [_ _]
                  tunnel: [w326 _] -> w319
                  tunnel: [w325 _] -> w318
                  frame False {
                    # "Not Canceled"
                    n207 = stacked-sequence {
                      tunnel: [w336 _] -> w326
                      tunnel: [w329 _] -> w325
                      tunnel: w324 -> [w327 _]
                      frame #0 {
                        n208 = local read "dir name"() -> (w333:string)
                        n209 = String To Path(string=w333) -> (path=w334:path)
                        n210 = Build Path(base path=w334, name or relative path=w327) -> (appended path=w335:path)
                        n211 = Path To String(path=w335) -> (string=w332:string)
                        n212 = call "util-path.vi"("append path (ie. folder\\filename.*)"=w332) -> ("error out"=w330:errorcluster, "SelectedPath"=w331:path)  [unwired: 6 in, 3 out]
                        n213 = Create Folder(path (use dialog)=w331, error in=w330) -> (cancelled=w328:bool, error out=w329:errorcluster)  [unwired: 1 in, 1 out]
                        n214 = Compound Arithmetic op=OR(w328, w329) -> (invert w336:bool)
                      }
                      frame #1 {
                        n215 = disable-structure shown="Disabled" {
                          disable-tunnel: [w349 _] -> _
                          disable-tunnel: [w348 _] -> _
                          frame Disabled {
                            n216 = local read "dir name"() -> (w340:string)
                            n217 = property on="SEC" class="Ring (strict)"() -> ("RingText.Text"=w339:string)  [unwired: 2 in, 2 out]
                            n218 = property on="SEC" class="Ring (strict)"() -> ("RingText.Text"=w345:string)  [unwired: 2 in, 2 out]
                            n219 = local read "dir name"() -> (w346:string)
                            n220 = String To Path(string=w346) -> (path=w347:path)
                            n221 = String To Path(string=w340) -> (path=w341:path)
                            n222 = Build Path(base path=w347, name or relative path=w345) -> (appended path=w344:path)
                            n223 = Build Path(base path=w341, name or relative path=w339) -> (appended path=w342:path)
                            n224 = Path To String(path=w344) -> (string=w343:string)
                            n225 = Path To String(path=w342) -> (string=w338:string)
                            n226 = call "util-path.vi"("append path (ie. folder\\filename.*)"=w343) -> ("error out"=w352:errorcluster, "SelectedPath"=w354:path)  [unwired: 6 in, 3 out]
                            n227 = call "util-path.vi"("append path (ie. folder\\filename.*)"=w338) -> ("error out"=w351:errorcluster, "SelectedPath"=w353:path)  [unwired: 6 in, 3 out]
                            n228 = Merge Errors(w352, w351) -> (w350:errorcluster)
                            n229 = Copy(8:w350, 10:w353, 11:w354) -> (0:w348:errorcluster, 1:w337:bool)  [unwired: 2 in, 1 out]
                            n230 = Compound Arithmetic op=OR(w337, w348) -> (invert w349:bool)
                          }
                          frame Enabled {
                          }
                        }
                      }
                    }
                  }
                  frame True {
                    # "Cancelled"
                  }
                }
              }
              frame Default {
              }
            }
          }
          event Panel Close? {
            n231 = event-data() -> ()  [unwired: 1 in, 1 out]
            n232 = property on="Data Changed?" class="Bool (strict)"() -> ("Value"=w357:bool)  [unwired: 2 in, 2 out]
            n233 = case shown="True" w357 {
              tunnel: [FALSE ("T button?") w360] -> _
              tunnel: [TRUE ("T button?") w361] -> w356
              frame False {
              }
              frame True {
                n234 = Two Button Dialog(message="Proceed without saving?") -> (T button?=w361:bool)  [unwired: 2 in]
                n235 = Not(x=w361) -> (.not. x?=w360:bool)
              }
            }
            n236 = event-data("Discard?"=TRUE) -> ()  [unwired: 1 in, 1 out]
          }
          event Timeout {
            n237 = event-data() -> ()  [unwired: 1 in, 3 out]
            n238 = global read "globals-engine.vi" "STOP"() -> (w363:bool)
          }
        }
        n239 = case shown="False" w50 {
          selector: w50 -> [_ w57]
          frame False {
          }
          frame True {
            n240 = property on="SEC Reload" class="Bool (strict)"("Val(Sgnl)"=w57) -> ()  [unwired: 2 in, 2 out]
          }
        }
        n241 = case shown="True" w49 {
          selector: w49 -> [_ w56]
          frame False {
          }
          frame True {
            n242 = property on="DEV Reload" class="Bool (strict)"("Val(Sgnl)"=w56) -> ()  [unwired: 2 in, 2 out]
          }
        }
        n243 = call <vilib>:"Simple Error Handler.vi"("type of dialog (OK msg:1)"=w51, "error in (no error)"=w52) -> ()  [unwired: 3 in, 5 out]
        "event counter" <- w53
      }
    }
    frame #2 {
      n244 = case shown="True" TRUE {
        frame False {
        }
        frame True {
          n245 = control-ref of="This VI"() -> (w366:refnum<vi>)
          n246 = property class="VI"(reference=w366, "FP.State"=T15."Closed" ("Front Panel Window:State")) -> ()  [unwired: 1 in, 2 out]
        }
      }
    }
  }
  n247 = disable-structure shown="Enabled" {
    frame Disabled {
    }
    frame Enabled {
    }
  }
  "dir name" <- w9
